vi "Configure Gauge Activation.vi"(6 "thresholds":cluster{"on":dbl, "off":dbl}, 7 "gauge":u16(ring)=1 items=["1"=1, "2"=2, "3"=3], 8 "error in (no error)":errorcluster, 9 "deactivation":u16(ring) items=["manual"=0, "self control"=1, "channel 1"=3, "channel 2"=4, "channel 3"=5], 10 "activation":u16(ring) items=["manual"=0, "hot start"=1, "channel 1"=3, "channel 2"=4, "channel 3"=5], 11 "VGC in":refnum<class "PL Inficon VGC.lvclass">) -> (0 "error out":errorcluster, 1 "deactivation":u16(ring) items=["manual"=0, "self control"=1, "channel 1"=3, "channel 2"=4, "channel 3"=5], 2 "activation":u16(ring) items=["manual"=0, "hot start"=1, "channel 1"=3, "channel 2"=4, "channel 3"=5], 3 "VGC out":refnum<class "PL Inficon VGC.lvclass">, 4 "thresholds":cluster{"on":dbl, "off":dbl})   [LabVIEW 2015, in "PL Inficon VGC.lvclass"]
doc: "Configures gauge activation."
uses:
  PL Inficon VGC.lvclass
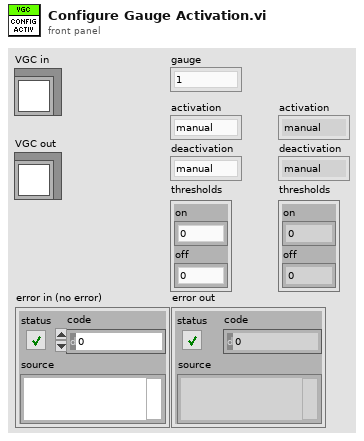
[diagram p1: front panel]
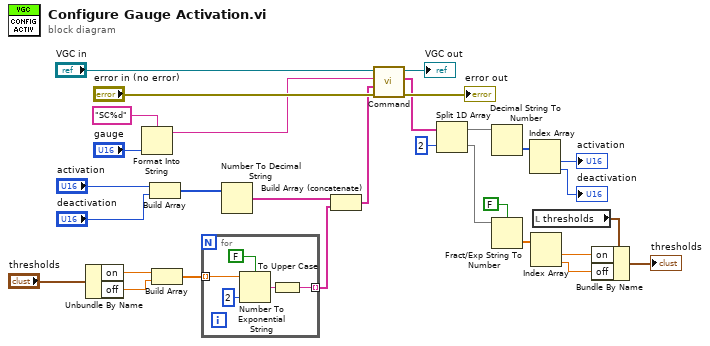
[diagram p0: block diagram]
diagram:
  n1 = Unbundle By Name("thresholds") -> ("on"=w6:dbl, "off"=w5:dbl)
  n2 = Format Into String(format string="SC%d", "gauge") -> (resulting string=w16:string)  [unwired: 2 in, 1 out]
  n3 = Build Array("activation", "deactivation") -> (w10:u16[])
  n4 = Build Array(w6, w5) -> (w12:dbl[])
  n5 = for {
    tunnel: w12 -> [w32] mode=indexing
    tunnel: [w31] -> w11 mode=indexing
    n6 = Number To Exponential String(number=w32, precision (6)=i16 2, 1:FALSE ("use system decimal point (T)")) -> (E-format string=w33:string)  [unwired: 1 in]
    n7 = To Upper Case(1:w33) -> (0:w31:string)
  }
  n8 = Number To Decimal String(number=w10) -> (decimal integer string=w19:string[])  [unwired: 1 in]
  n9 = Build Array (concatenate)(w19, w11) -> (w15:string[])
  n10 = call "Command.vi"("error in (no error)"="error in (no error)", "parameters"=w15, "command"=w16, "VGC in"="VGC in") -> ("error out"=→"error out":errorcluster, "response data"=w25:string[], "VGC out"=→"VGC out":refnum<class "PL Inficon VGC.lvclass">)  [unwired: 5 in]
  n11 = Split 1D Array(array=w25, index=2) -> (first subarray=w23:string[], second subarray=w22:string[])
  n12 = Decimal String To Number(string=w23) -> (number=w14:i32[])  [unwired: 2 in, 1 out]
  n13 = Fract/Exp String To Number(use system decimal point (T)=FALSE, string=w22) -> (number=w21:dbl[])  [unwired: 2 in, 1 out]
  n14 = Index Array(array=w14) -> (element #1=→"activation":i32, element #2=→"deactivation":i32)  [unwired: 2 in]
  n15 = Index Array(array=w21) -> (element #1=w3:dbl, element #2=w2:dbl)  [unwired: 2 in]
  n16 = local read "thresholds"() -> (w4:cluster{"on":dbl, "off":dbl})
  n17 = Bundle By Name(cluster=w4, "on"=w3, "off"=w2) -> (→"thresholds":cluster{"on":dbl, "off":dbl})
